vi "set_config_cluster.vi"(8 "error in (no error)":errorcluster, 10 "config cluster variant":variant, 11 "ImagingModeDL090923Scaffold in":refnum<class "ImagingModeDL090923Scaffold.lvclass">) -> (0 "error out":errorcluster, 3 "ImagingModeDL090923Scaffold out":refnum<class "ImagingModeDL090923Scaffold.lvclass">)   [LabVIEW 2010, in "ImagingModeDL090923Scaffold.lvclass"]
uses:
  ImagingModeDL090923Scaffold.lvclass
  ImagingModeDL090923Scaffold.lvclass/ImagingModeDL090923Scaffold.ctl
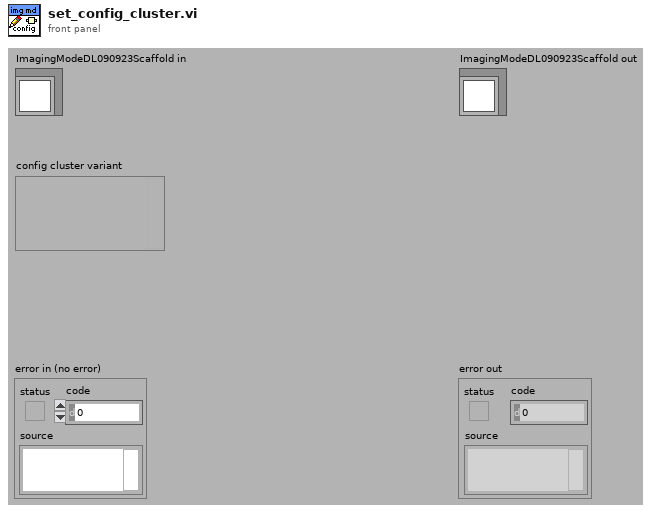
[diagram p1: front panel]
types:
  T1 = typedef "ImagingModeDL090923Scaffold.lvclass/config_data_cluster.ctl" = cluster{"Instrument":T2, "Trajectory":T2, "ScanHead":T2, "DAQ":T2, "ImageAssembler":T2, "DataCollection":T2, "Display":T2, "Analyser":T2, "Stimulator":T2, "Trajectory-to-ImageAssembler adapter path":string, "LSID (cluster)":T4}
  T2 = typedef "ImagingModeDL090923Scaffold.lvclass/component_specification_cluster.ctl" = cluster{"specification":T3, "adapter path":string}
  T3 = typedef "plugin_specification.ctl" = cluster{"class path":string, "configuration":string, "label":string, "settings name":string}
  T4 = typedef "LSID_cluster.ctl" = cluster{"identifier":string, "revision":i32}
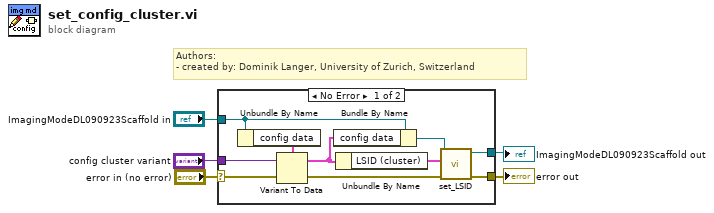
[diagram p0: block diagram]
diagram:
  # "Authors: \n- created by: Dominik Langer, University of Zurich, Switzerland"
  n1 = case shown="No Error" "error in (no error)" {
    selector: "error in (no error)" -> [w9 w17]
    tunnel: [w15 w17] -> w2
    tunnel: [w14 w16] -> w1
    tunnel: "ImagingModeDL090923Scaffold in" -> [w7 w16]
    tunnel: "config cluster variant" -> [w10 _]
    frame No Error {
      n2 = Unbundle By Name(w7) -> ("config data"=w11:T1)
      n3 = Variant To Data(error in=w9, Variant=w10, type=w11) -> (error out=w8:errorcluster, data=w13:T1)
      n4 = Bundle By Name(cluster=w7, "config data"=w13) -> (w6:refnum<class "ImagingModeDL090923Scaffold.lvclass">)
      n5 = Unbundle By Name(w13) -> ("LSID (cluster)"=w12:T4)
      n6 = call-dynamic "set_LSID.vi"("error in (no error)"=w8, "LSID"=w12, "GenericPlugin in"=w6) -> ("error out"=w15:errorcluster, "GenericPlugin out"=w14:refnum<class "ImagingModeDL090923Scaffold.lvclass">)  [unwired: 7 in]
    }
    frame Error {
    }
  }
  "error out" <- w2
  "ImagingModeDL090923Scaffold out" <- w1
